vi "Initialize.vi"(8 "error in":errorcluster, 11 "Plugin in":refnum<class "Configure Visa Device Channels.lvclass">) -> (0 "error out":errorcluster, 3 "Plugin out":refnum<class "Configure Visa Device Channels.lvclass">)   [LabVIEW 2026, in "Configure Visa Device Channels.lvlib" / "Configure Visa Device Channels.lvclass"]
uses:
  Configure Visa Device Channels.lvclass
  <vilib>/FlexLogger/SDK/PluginSDK.lvlibp/PEFClasses/SDK/Producer Channel/Producer Channel.lvclass
  <vilib>/FlexLogger/SDK/PluginSDK.lvlibp/PEFClasses/SDK/Plugin/ParameterAccess/Write String.vi
  <vilib>/FlexLogger/SDK/PluginSDK.lvlibp/PEFClasses/SDK/Plugin/ParameterAccess/Write I32.vi
  <vilib>/FlexLogger/SDK/PluginSDK.lvlibp/PEFClasses/SDK/Producer Channel/Create Producer Channel_v2.vi
  <vilib>/FlexLogger/SDK/PluginSDK.lvlibp/PEFClasses/SDK/Channel/ParameterAccess/Write String.vi
  <vilib>/FlexLogger/SDK/PluginSDK.lvlibp/PEFClasses/SDK/Channel/ParameterAccess/Write DBL.vi
  <vilib>/FlexLogger/SDK/PluginSDK.lvlibp/PEFClasses/SDK/Plugin/Plugin.lvclass
  <vilib>/FlexLogger/SDK/PluginSDK.lvlibp
  <vilib>/FlexLogger/SDK/PluginSDK.lvlibp/PEFClasses/SDK/Channel/Channel.lvclass
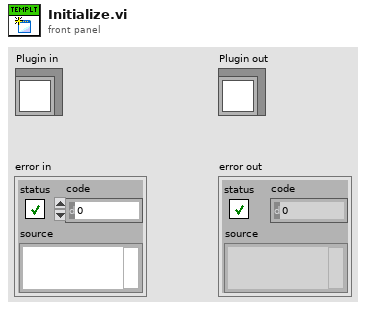
[diagram p1: front panel]
types:
  T1 = cluster{"Timing Method":enum16{"Periodic", "Immediate", "On Data Ready", "Triggered"}, "Timing Period (ms)":i32}
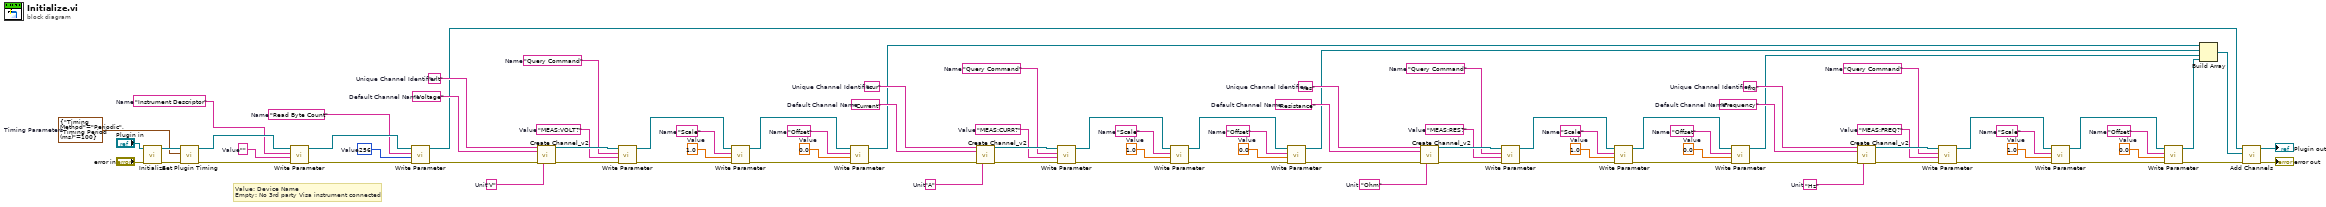
[diagram p0: block diagram]
diagram:
  w11 = 0.0  # Value
  w12 = "Offset"  # Name
  w15 = 1.0  # Value
  w16 = "Scale"  # Name
  w19 = "MEAS:FREQ?"  # Value
  w20 = "Query Command"  # Name
  w22 = "Hz"  # Unit
  w24 = "Frequency"  # Default Channel Name
  w25 = "frq"  # Unique Channel Identifier
  w27 = 0.0  # Value
  w28 = "Offset"  # Name
  w31 = 1.0  # Value
  w32 = "Scale"  # Name
  w35 = "MEAS:RES?"  # Value
  w36 = "Query Command"  # Name
  w38 = "Ohm"  # Unit
  w40 = "Resistance"  # Default Channel Name
  w41 = "res"  # Unique Channel Identifier
  w43 = 0.0  # Value
  w44 = "Offset"  # Name
  w47 = 1.0  # Value
  w48 = "Scale"  # Name
  w51 = "MEAS:CURR?"  # Value
  w52 = "Query Command"  # Name
  w54 = "A"  # Unit
  w56 = "Current"  # Default Channel Name
  w57 = "cur"  # Unique Channel Identifier
  w59 = 0.0  # Value
  w60 = "Offset"  # Name
  w63 = 1.0  # Value
  w64 = "Scale"  # Name
  w67 = "MEAS:VOLT?"  # Value
  w68 = "Query Command"  # Name
  w70 = "V"  # Unit
  w72 = "Voltage"  # Default Channel Name
  w73 = "vlt"  # Unique Channel Identifier
  w75 = 256  # Value
  w76 = "Read Byte Count"  # Name
  w79 = ""  # Value
  w80 = "Instrument Descriptor"  # Name
  w83 = T1 {"Timing Method"=enum."Periodic", "Timing Period (ms)"=100}  # Timing Parameters
  # "Value: Device Name\nEmpty: No 3rd party Visa instrument connected"
  n1 = call-parent "Initialize.vi"("error in (no error)"="error in", "Plugin in"="Plugin in") -> ("error out"=w82:errorcluster, "Plugin out"=w84:refnum<class "Configure Visa Device Channels.lvclass">)  [unwired: 8 in]
  n2 = call <vilib>:"Set Plugin Timing.vi"("error in (no error)"=w82, "Timing Parameters"=w83, "Plugin in"=w84) -> ("error out"=w78:errorcluster, "Plugin out"=w81:refnum<class "Configure Visa Device Channels.lvclass">)  [unwired: 7 in]
  n3 = call-poly <vilib>:"Write Parameter.vi"("error in (no error)"=w78, "Value"=w79, "Name"=w80, "Plugin in"=w81) -> ("error out"=w74:errorcluster, "Plugin out"=w77:refnum<class "Configure Visa Device Channels.lvclass">)  [unwired: 6 in]
  n4 = call-poly <vilib>:"Write Parameter.vi"("error in (no error)"=w74, "Value"=w75, "Name"=w76, "Plugin in"=w77) -> ("error out"=w71:errorcluster, "Plugin out"=w5:refnum<class "Configure Visa Device Channels.lvclass">)  [unwired: 6 in]
  n5 = call-poly <vilib>:"Create Channel_v2.vi"("Unique Channel Identifier"=w73, "Default Channel Name"=w72, "error in (no error)"=w71, "Unit"=w70) -> ("Producer Channel"=w69:refnum<class "Producer Channel.lvclass">, "error out"=w66:errorcluster)  [unwired: 10 in]
  n6 = call-poly <vilib>:"Write Parameter.vi"("error in (no error)"=w66, "Value"=w67, "Name"=w68, "Channel in"=w69) -> ("error out"=w62:errorcluster, "Channel out"=w65:refnum<class "Producer Channel.lvclass">)  [unwired: 6 in]
  n7 = call-poly <vilib>:"Write Parameter.vi"("error in (no error)"=w62, "Value"=w63, "Name"=w64, "Channel in"=w65) -> ("error out"=w58:errorcluster, "Channel out"=w61:refnum<class "Producer Channel.lvclass">)  [unwired: 6 in]
  n8 = call-poly <vilib>:"Write Parameter.vi"("error in (no error)"=w58, "Value"=w59, "Name"=w60, "Channel in"=w61) -> ("error out"=w55:errorcluster, "Channel out"=w9:refnum<class "Producer Channel.lvclass">)  [unwired: 6 in]
  n9 = call-poly <vilib>:"Create Channel_v2.vi"("Unique Channel Identifier"=w57, "Default Channel Name"=w56, "error in (no error)"=w55, "Unit"=w54) -> ("Producer Channel"=w53:refnum<class "Producer Channel.lvclass">, "error out"=w50:errorcluster)  [unwired: 10 in]
  n10 = call-poly <vilib>:"Write Parameter.vi"("error in (no error)"=w50, "Value"=w51, "Name"=w52, "Channel in"=w53) -> ("error out"=w46:errorcluster, "Channel out"=w49:refnum<class "Producer Channel.lvclass">)  [unwired: 6 in]
  n11 = call-poly <vilib>:"Write Parameter.vi"("error in (no error)"=w46, "Value"=w47, "Name"=w48, "Channel in"=w49) -> ("error out"=w42:errorcluster, "Channel out"=w45:refnum<class "Producer Channel.lvclass">)  [unwired: 6 in]
  n12 = call-poly <vilib>:"Write Parameter.vi"("error in (no error)"=w42, "Value"=w43, "Name"=w44, "Channel in"=w45) -> ("error out"=w39:errorcluster, "Channel out"=w8:refnum<class "Producer Channel.lvclass">)  [unwired: 6 in]
  n13 = call-poly <vilib>:"Create Channel_v2.vi"("Unique Channel Identifier"=w41, "Default Channel Name"=w40, "error in (no error)"=w39, "Unit"=w38) -> ("Producer Channel"=w37:refnum<class "Producer Channel.lvclass">, "error out"=w34:errorcluster)  [unwired: 10 in]
  n14 = call-poly <vilib>:"Write Parameter.vi"("error in (no error)"=w34, "Value"=w35, "Name"=w36, "Channel in"=w37) -> ("error out"=w30:errorcluster, "Channel out"=w33:refnum<class "Producer Channel.lvclass">)  [unwired: 6 in]
  n15 = call-poly <vilib>:"Write Parameter.vi"("error in (no error)"=w30, "Value"=w31, "Name"=w32, "Channel in"=w33) -> ("error out"=w26:errorcluster, "Channel out"=w29:refnum<class "Producer Channel.lvclass">)  [unwired: 6 in]
  n16 = call-poly <vilib>:"Write Parameter.vi"("error in (no error)"=w26, "Value"=w27, "Name"=w28, "Channel in"=w29) -> ("error out"=w23:errorcluster, "Channel out"=w7:refnum<class "Producer Channel.lvclass">)  [unwired: 6 in]
  n17 = call-poly <vilib>:"Create Channel_v2.vi"("Unique Channel Identifier"=w25, "Default Channel Name"=w24, "error in (no error)"=w23, "Unit"=w22) -> ("Producer Channel"=w21:refnum<class "Producer Channel.lvclass">, "error out"=w18:errorcluster)  [unwired: 10 in]
  n18 = call-poly <vilib>:"Write Parameter.vi"("error in (no error)"=w18, "Value"=w19, "Name"=w20, "Channel in"=w21) -> ("error out"=w14:errorcluster, "Channel out"=w17:refnum<class "Producer Channel.lvclass">)  [unwired: 6 in]
  n19 = call-poly <vilib>:"Write Parameter.vi"("error in (no error)"=w14, "Value"=w15, "Name"=w16, "Channel in"=w17) -> ("error out"=w10:errorcluster, "Channel out"=w13:refnum<class "Producer Channel.lvclass">)  [unwired: 6 in]
  n20 = call-poly <vilib>:"Write Parameter.vi"("error in (no error)"=w10, "Value"=w11, "Name"=w12, "Channel in"=w13) -> ("error out"=w3:errorcluster, "Channel out"=w6:refnum<class "Producer Channel.lvclass">)  [unwired: 6 in]
  n21 = Build Array(w9, w8, w7, w6) -> (w4:refnum<class "Producer Channel.lvclass">[])
  n22 = call <vilib>:"Add Channels.vi"("error in (no error)"=w3, "Channels"=w4, "Plugin in"=w5) -> ("error out"=→"error out":errorcluster, "Plugin out"=→"Plugin out":refnum<class "Configure Visa Device Channels.lvclass">)  [unwired: 7 in]
